vi "Main_control.vi"() -> ()   [LabVIEW 2019]
uses:
  F710PackedLibrary.lvlibp/F710.ctl
  F710PackedLibrary.lvlibp/stick.ctl
  F710PackedLibrary.lvlibp/gamepadF710.lvclass
  <vilib>/Platform/TimedLoop/XDataNode/timing_clust.ctl
  <vilib>/Platform/TimedLoop/XDataNode/nitl_modes.ctl
  <vilib>/Platform/TimedLoop/XDataNode/wakeup.ctl
  <vilib>/platform/TimedLoop/XDataNode/XDataNode.xnode
  KNRm_ReMi_OS6_436Motor.lvlibp
  <vilib>/ptbypt/NI_PtbyPt.lvlib
  <vilib>/Platform/TimedLoop/XDataNode/XDNodeRunTimeDep.lvlib
  F710PackedLibrary.lvlibp
panel:
  out "F710 button info.start":bool
  out "start":bool
  out "F710":T1
  out "coerced(x)":dbl[](array[numeric])
  out "Y":dbl
  out "turn":dbl
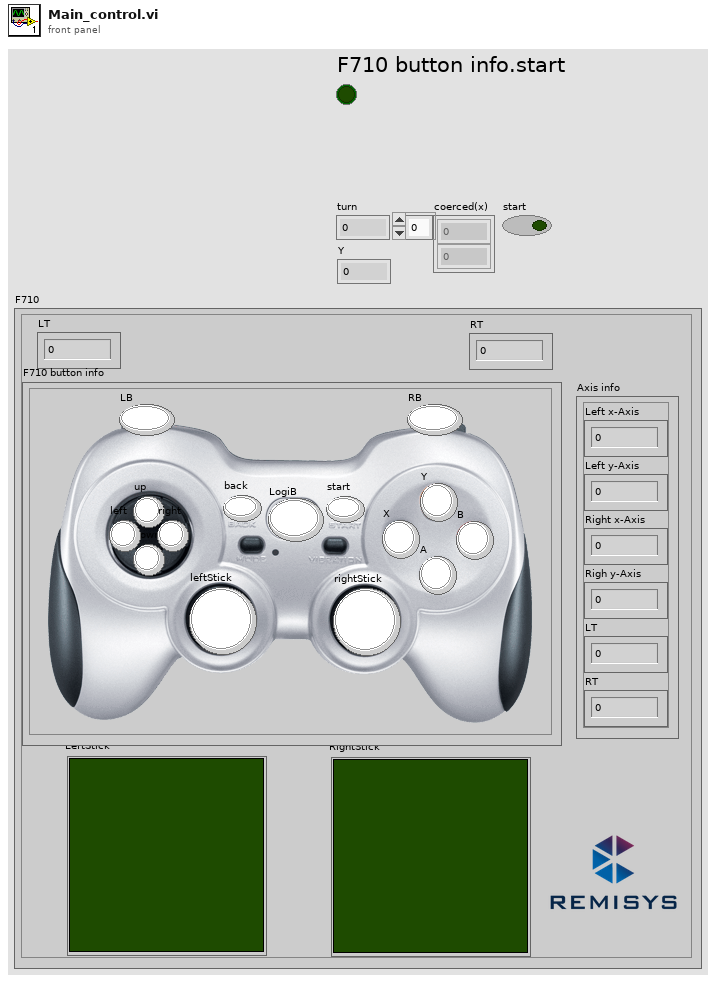
[diagram p1: front panel]
types:
  T1 = typedef "F710PackedLibrary.lvlibp/F710.ctl" = cluster{"RT":u8, "LT":u8, "RightStick":T2, "LeftStick":T2, "Axis info":cluster{"Left x-Axis":i8, "Left y-Axis":i8, "Right x-Axis":i8, "Righ y-Axis":i8, "LT":u8, "RT":u8}, "F710 button info":cluster{"RB":bool, "LB":bool, "rightStick":bool, "leftStick":bool, "start":bool, "back":bool, "right":bool, "left":bool, "down":bool, "up":bool, "Y":bool, "X":bool, "B":bool, "A":bool, "LogiB":bool}}
  T2 = typedef "F710PackedLibrary.lvlibp/stick.ctl" = cluster{"X":dbl, "Y":dbl}[]
  T3 = typedef "XDNodeRunTimeDep.lvlib/timing_clust.ctl" = cluster{"Expected End [f-1]":u64, "Actual End [f-1]":u64, "Finished Late? [f-1]":bool, "Expected End [i-1]":u64, "Actual End [i-1]":u64, "Finished Late? [i-1]":bool, "Expected Start [i]":u64, "Actual Start [i]":u64, "Expected Start [f]":u64, "Actual Start [f]":u64, "Source Name":string, "Structure Name":string, "Period":i64, "Deadline":i64, "Offset":i64, "Start":i64, "Priority":i32, "Timeout":i32, "Mode":T4, "Wakeup Reason":T5, "Error":errorcluster, "Source Type":string, "Secondary Source Type":string, "Global End Time":u64, "Global Start Time":u64, "Frame Duration":u64, "Iteration Duration":u64, "Assigned CPU":i32, "I/O Scan Engine Mode":u32}
  T4 = typedef "XDNodeRunTimeDep.lvlib/nitl_modes.ctl" = enum32{"No Change", "Process missed periods, maintain original phase", "Discard missed periods, maintain original phase", "Process missed periods, ignore original phase", "Discard missed periods, ignore original phase"}
  T5 = typedef "XDNodeRunTimeDep.lvlib/wakeup.ctl" = enum32{"Normal", "Aborted", "Asynchronous wakeup", "Timing source error", "Timed loop error", "Timeout"}
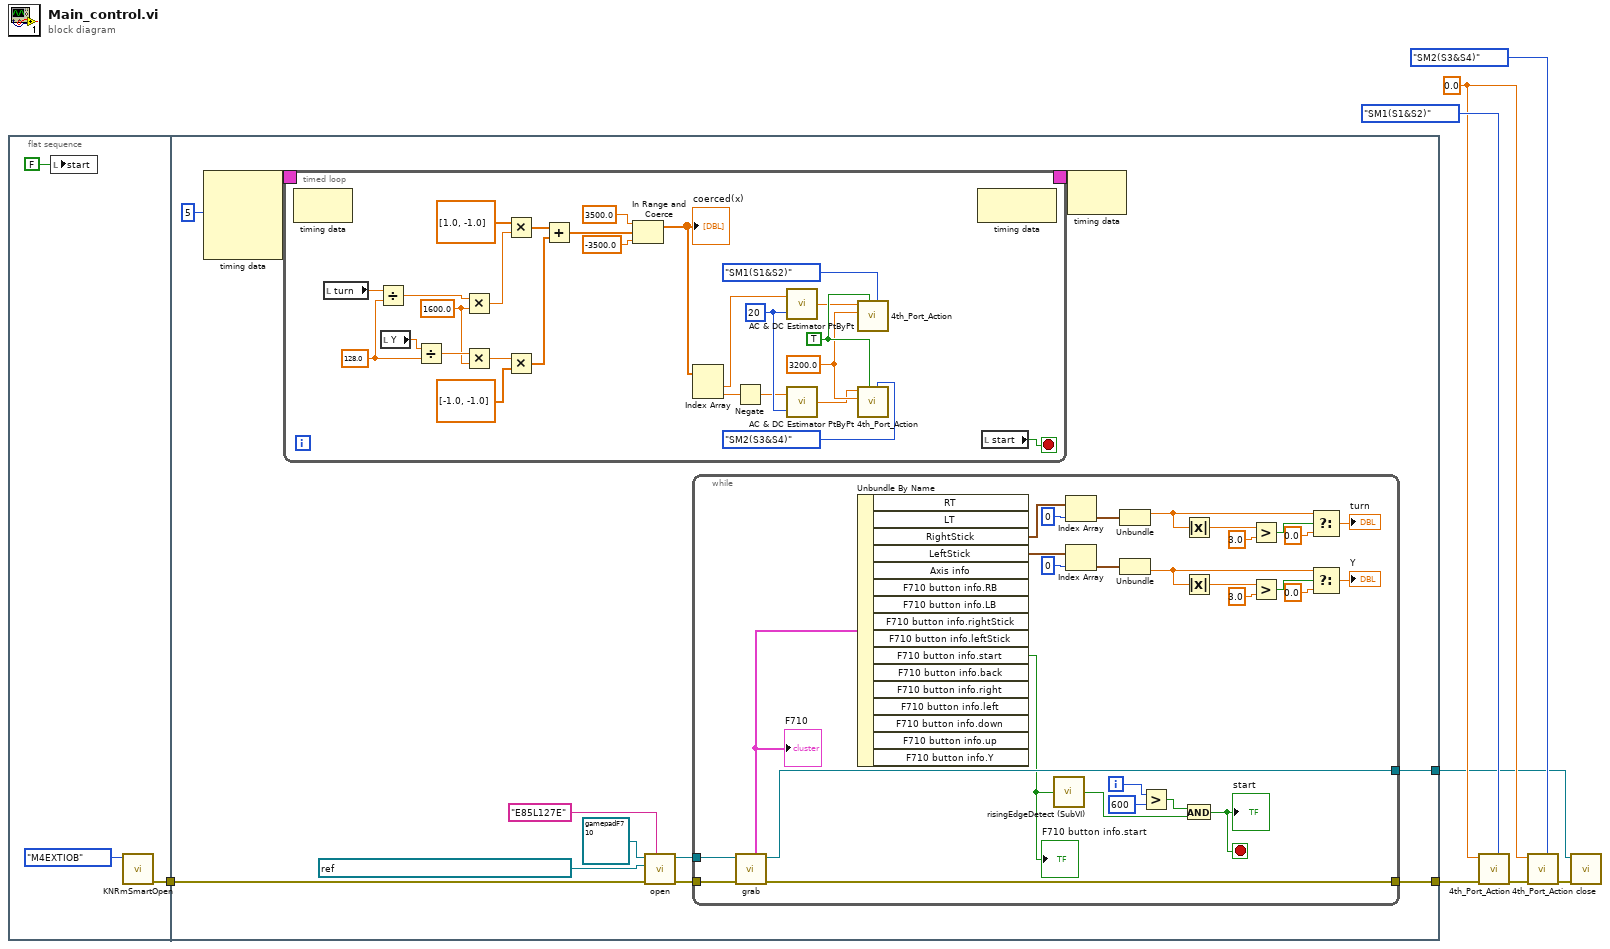
[diagram p0: block diagram]
diagram:
  w4 = 0.0 ("vel(deg/sec)")
  n1 = flat-sequence {
    tunnel: [w10] -> w8
    tunnel: w8 -> [w18]
    tunnel: [w17] -> w3
    tunnel: [w15] -> w2
    frame #0 {
      n2 = local write "start"(FALSE ("stop")) -> ()
      n3 = call "KNRmSmartOpen.vi"("INI FPGA MODE"=enum16{"Original", "M4EXTIOB"}."M4EXTIOB") -> ("error out"=w10:errorcluster)  [unwired: 7 in, 3 out]
    }
    frame #1 {
      n4 = node-c288(i64 5 ("Period")) -> (w14:T3)  [unwired: 3 in]
      n5 = timed-loop {
        timing: w14 -> [_]
        timing-out: [_] -> w13
        stop <- w29 stop-if-true
        w26 = 20 ("sample length")
        w25 = 3200.0 ("step")
        w31 = TRUE ("EN")
        w39 = 1600.0 ("y")
        w38 = 128.0 ("y")
        n6 = node-c288() -> ()  [unwired: 1 in, 1 out]
        n7 = local read "turn"() -> (w49:dbl)
        n8 = Divide(x=w49, y=w38) -> (x/y=w48:dbl)
        n9 = local read "Y"() -> (w46:dbl)
        n10 = Divide(x=w46, y=w38) -> (x/y=w47:dbl)
        n11 = Multiply(x=w48, y=w39) -> (x*y=w45:dbl)
        n12 = Multiply(x=w47, y=w39) -> (x*y=w43:dbl)
        n13 = Multiply(x=dbl[] [1.0, -1.0], y=w45) -> (x*y=w41:dbl[])
        n14 = Multiply(x=w43, y=dbl[] [-1.0, -1.0]) -> (x*y=w40:dbl[])
        n15 = Add(x=w41, y=w40) -> (x+y=w37:dbl[])
        n16 = In Range and Coerce(upper limit=3500.0 ("y"), x=w37, lower limit=-3500.0 ("y")) -> (coerced(x)=w33:dbl[])  [unwired: 1 out]
        "coerced(x)" <- w33
        n17 = Index Array(array=w33) -> (element #1=w28:dbl, element #2=w30:dbl)  [unwired: 2 in]
        n18 = Negate(x=w30) -> (-x=w24:dbl)
        n19 = call <vilib>:"AC & DC Estimator PtByPt.vi"("signal"=w28, "sample length"=w26) -> ("DC estimate (V)"=w27:dbl)  [unwired: 1 in, 2 out]
        n20 = call <vilib>:"AC & DC Estimator PtByPt.vi"("signal"=w24, "sample length"=w26) -> ("DC estimate (V)"=w23:dbl)  [unwired: 1 in, 2 out]
        n21 = call "4th_Port_Action.vi"("Port"=enum16{"SM1(S1&S2)", "SM2(S3&S4)", "SM3(S5&S6)"}."SM1(S1&S2)", "EN"=w31, "step"=w25, "vel(deg/sec)"=w27) -> ()  [unwired: 5 in, 3 out]
        n22 = call "4th_Port_Action.vi"("Port"=enum16{"SM1(S1&S2)", "SM2(S3&S4)", "SM3(S5&S6)"}."SM2(S3&S4)", "EN"=w31, "step"=w25, "vel(deg/sec)"=w23) -> ()  [unwired: 5 in, 3 out]
        n23 = node-c288() -> ()  [unwired: 1 in, 1 out]
        n24 = local read "start"() -> (w29:bool)
      }
      n25 = call "open.vi"("INPUT S/N"="E85L127E", "error in (no error)"=w18, "VISA resource name"=refnum<visa-resource-name> "USB0::0x046D::0xC21F::9BD89EBC::RAW", "gamepadF710 in"=refnum<class "gamepadF710.lvclass"> refnum ("F710PackedLibrary.lvlibp:gamepadF710.lvclass")) -> ("error out"=w16:errorcluster, "gamepadF710 out"=w20:refnum<class "gamepadF710.lvclass">)  [unwired: 5 in, 1 out]
      n26 = while {
        tunnel: w20 -> [w84]
        tunnel: [w83] -> w17
        tunnel: w16 -> [w64]
        tunnel: [w63] -> w15
        i -> [w60]
        stop <- w56 stop-if-true
        n27 = call "grab.vi"("error in (no error)"=w64, "gamepadF710 in"=w84) -> ("error out"=w63:errorcluster, "gamepadF710 out"=w83:refnum<class "gamepadF710.lvclass">, "F710"=w61:T1)  [unwired: 6 in]
        "F710" <- w61
        n28 = Unbundle By Name(w61) -> ("RightStick"=w82:T2, "LeftStick"=w77:T2, "F710 button info.start"=w62:bool)  [unwired: 13 out]
        "F710 button info.start" <- w62
        n29 = call "risingEdgeDetect (SubVI).vi"("input"=w62) -> ("output"=w57:bool)
        n30 = Index Array(array=w82, index=0) -> (element=w80:cluster{"X":dbl, "Y":dbl})
        n31 = Index Array(array=w77, index=0) -> (element=w79:cluster{"X":dbl, "Y":dbl})
        n32 = Unbundle(w80) -> ("X"=w71:dbl)  [unwired: 1 out]
        n33 = Unbundle(w79) -> ("Y"=w66:dbl)  [unwired: 1 out]
        n34 = Greater?(x=w60, y=600) -> (0:w58:bool)
        n35 = Absolute Value(x=w71) -> (abs(x)=w76:dbl)
        n36 = Absolute Value(x=w66) -> (abs(x)=w67:dbl)
        n37 = And(x=w58, y=w57) -> (x .and. y?=w56:bool)
        "start" <- w56
        n38 = Greater?(x=w76, y=3.0) -> (0:w74:bool)
        n39 = Greater?(x=w67, y=3.0) -> (0:w69:bool)
        n40 = Select(t=w71, s=w74, f=0.0) -> (s? t:f=→"turn":dbl)
        n41 = Select(t=w66, s=w69, f=0.0) -> (s? t:f=→"Y":dbl)
      }
      n42 = node-c288(w13) -> ()  [unwired: 1 out]
    }
  }
  n43 = call "4th_Port_Action.vi"("Port"=enum16{"SM1(S1&S2)", "SM2(S3&S4)", "SM3(S5&S6)"}."SM1(S1&S2)", "error in"=w2, "vel(deg/sec)"=w4) -> ("error out"=w5:errorcluster)  [unwired: 6 in, 2 out]
  n44 = call "4th_Port_Action.vi"("Port"=enum16{"SM1(S1&S2)", "SM2(S3&S4)", "SM3(S5&S6)"}."SM2(S3&S4)", "error in"=w5, "vel(deg/sec)"=w4) -> ("error out"=w1:errorcluster)  [unwired: 6 in, 2 out]
  n45 = call "close.vi"("error in (no error)"=w1, "gamepadF710 in"=w3) -> ()  [unwired: 8 in, 2 out]
